vi "test vi.vi"() -> ()   [LabVIEW 2016]
uses:
  JSON Helper/Parsing/Parse Value.vi
  JSON Helper/JSON Value.lvclass
panel:
  in  "JSON String":string="{\n        \"description\": \"the description of the test case\",\n        \"schema\": {\"the schema that should\" : \"be validated against\"},\n        \"tests\": [\n            {\n                \"description\": \"a specific test of a valid instance\",\n                \"data\": \"the instance\",\n                \"valid\": true\n            },\n            {\n                \"description\": \"another specific test this time, invalid\",\n                \"data\": 15,\n                \"valid\": false\n            }\n        ]\n    }"
  out "String":string
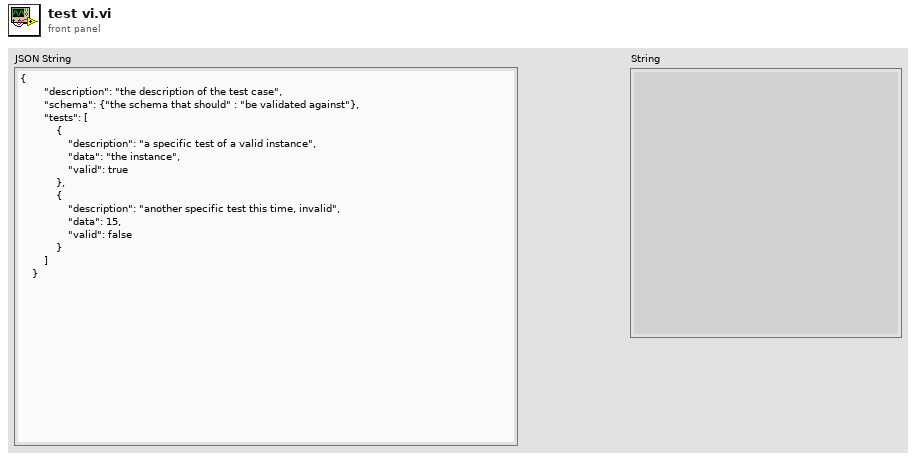
[diagram p1: front panel]
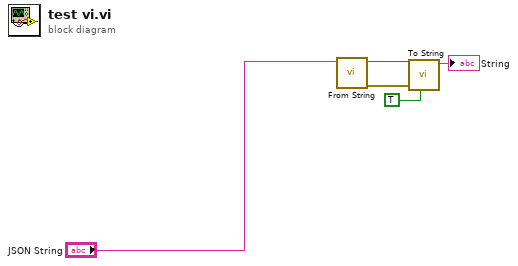
[diagram p0: block diagram]
diagram:
  n1 = call "From String.vi"("JSON String"="JSON String") -> ("error out"=w3:errorcluster, "JSON Value out"=w4:refnum<class "JSON Value.lvclass">)  [unwired: 9 in]
  n2 = call "To String.vi"("pretty print? (T)"=TRUE, "error in (no error)"=w3, "JSON Value in"=w4) -> ("String"=→"String":string)  [unwired: 7 in, 1 out]
